vi "cluster_inside_cluster_property.vi"() -> ()   [LabVIEW 2017]
panel:
  in  "Array":bool[](array[boolean])=[TRUE, TRUE, FALSE, TRUE, FALSE]
  out "Controls[]":refnum<vi>[](array[refnum])
  in  "Machine 10":T1
  # "Communication"
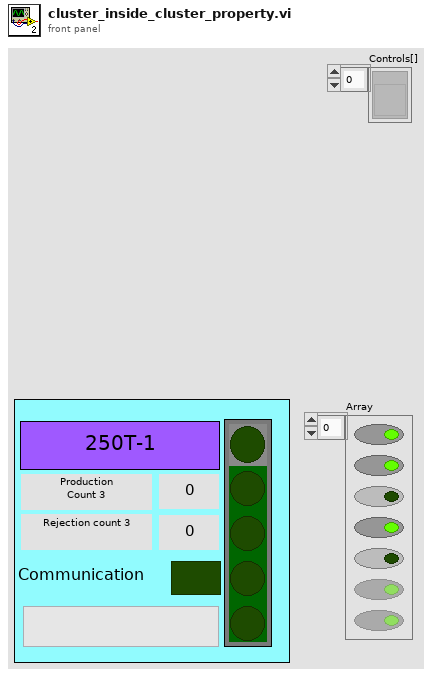
[diagram p1: front panel]
types:
  T1 = cluster{"Status 10":cluster{"S":bool, "l":bool, "M":bool, "Q":bool, "P":bool}, "Station 3":bool, "Production\nCount 3":i32, "Rejection count 3":i32, "String Indicator 3":bool, "Product code 10":string}
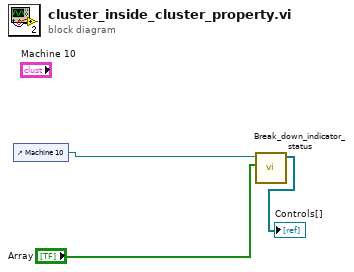
[diagram p0: block diagram]
diagram:
  n1 = control-ref of="Machine 10"() -> (w2:refnum<vi>)
  n2 = call "Break_down_indicator_status.vi"("Array"="Array", "Cluster in"=w2) -> ("Controls[]"=→"Controls[]":refnum<vi>[])  [unwired: 9 in]
